vi "获取X轴信息.vi"(10 "错误输入（无错误）":errorcluster, 11 "VISA资源名称":refnum<visa-resource-name>) -> (1 "错误输出":errorcluster, 2 "VISA资源名称输出":refnum<visa-resource-name>, 4 "XZEro":dbl, 5 "DeltX":dbl, 6 "XUNit":string, 7 "示波器刻度":dbl, 9 "坐标偏移量":dbl)   [LabVIEW 2017]
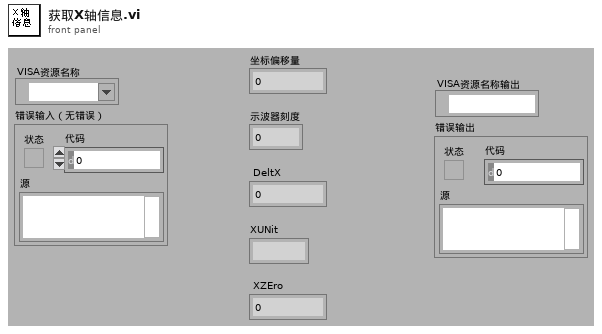
[diagram p1: front panel]
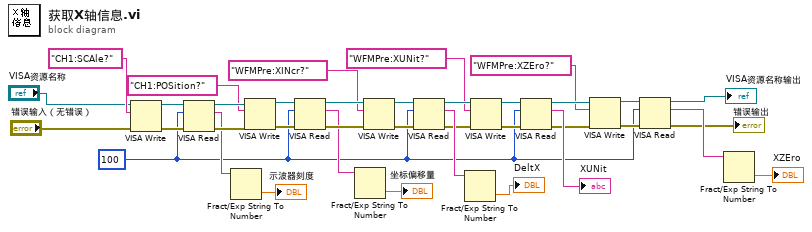
[diagram p0: block diagram]
diagram:
  w6 = u32 100 ("字节总数")
  n1 = VISA Write(VISA resource name="VISA资源名称", write buffer="CH1:SCAle?" ("string to write"), error in (no error)="错误输入（无错误）") -> (VISA resource name out=w37:refnum<visa-resource-name>, error out=w36:errorcluster)  [unwired: 1 out]
  n2 = VISA Read(VISA resource name=w37, byte count=w6, error in (no error)=w36) -> (VISA resource name out=w32:refnum<visa-resource-name>, read buffer=w29:string, error out=w31:errorcluster)  [unwired: 1 out]
  n3 = Fract/Exp String To Number(string=w29) -> (number=→"示波器刻度":dbl)  [unwired: 3 in, 1 out]
  n4 = VISA Write(VISA resource name=w32, write buffer="CH1:POSition?" ("string to write"), error in (no error)=w31) -> (VISA resource name out=w34:refnum<visa-resource-name>, error out=w33:errorcluster)  [unwired: 1 out]
  n5 = VISA Read(VISA resource name=w34, byte count=w6, error in (no error)=w33) -> (VISA resource name out=w24:refnum<visa-resource-name>, read buffer=w21:string, error out=w23:errorcluster)  [unwired: 1 out]
  n6 = Fract/Exp String To Number(string=w21) -> (number=→"坐标偏移量":dbl)  [unwired: 3 in, 1 out]
  n7 = VISA Write(VISA resource name=w24, write buffer="WFMPre:XINcr?" ("写入缓冲区"), error in (no error)=w23) -> (VISA resource name out=w26:refnum<visa-resource-name>, error out=w25:errorcluster)  [unwired: 1 out]
  n8 = VISA Read(VISA resource name=w26, byte count=w6, error in (no error)=w25) -> (VISA resource name out=w17:refnum<visa-resource-name>, read buffer=w20:string, error out=w16:errorcluster)  [unwired: 1 out]
  n9 = Fract/Exp String To Number(string=w20) -> (number=→"DeltX":dbl)  [unwired: 3 in, 1 out]
  n10 = VISA Write(VISA resource name=w17, write buffer="WFMPre:XUNit?" ("写入缓冲区"), error in (no error)=w16) -> (VISA resource name out=w19:refnum<visa-resource-name>, error out=w18:errorcluster)  [unwired: 1 out]
  n11 = VISA Read(VISA resource name=w19, byte count=w6, error in (no error)=w18) -> (VISA resource name out=w11:refnum<visa-resource-name>, read buffer=→"XUNit":string, error out=w10:errorcluster)  [unwired: 1 out]
  n12 = VISA Write(VISA resource name=w11, write buffer="WFMPre:XZEro?" ("写入缓冲区"), error in (no error)=w10) -> (VISA resource name out=w13:refnum<visa-resource-name>, error out=w12:errorcluster)  [unwired: 1 out]
  n13 = VISA Read(VISA resource name=w13, byte count=w6, error in (no error)=w12) -> (VISA resource name out=→"VISA资源名称输出":refnum<visa-resource-name>, read buffer=w7:string, error out=→"错误输出":errorcluster)  [unwired: 1 out]
  n14 = Fract/Exp String To Number(string=w7) -> (number=→"XZEro":dbl)  [unwired: 3 in, 1 out]
